vi "Read Provided Interface.vi"(8 "error in (no error)":errorcluster, 11 "instrument in":refnum<class "Instrument.lvclass">) -> (0 "error out":errorcluster, 2 "provided interface":string, 3 "instrument out":refnum<class "Instrument.lvclass">)   [LabVIEW 2020, in "MeasurementLink Instrument.lvlib" / "Instrument.lvclass"]
doc: "Returns the provided interface that will be used to query the MeasurmentLink Discovery Service for the address and port of the instrument's gRPC server. If your instrument does not use a gRPC server then you do not have to implement this VI."
uses:
  Instrument.lvclass
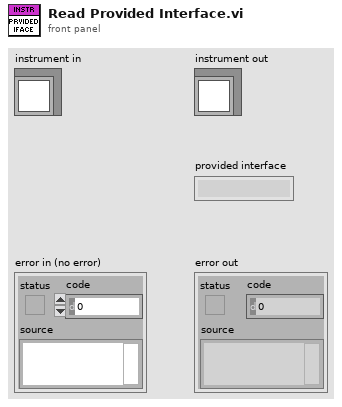
[diagram p1: front panel]
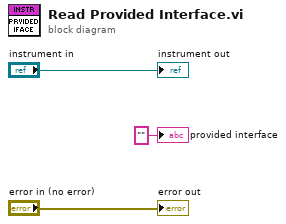
[diagram p0: block diagram]
diagram:
  "error out" <- "error in (no error)"
  "instrument out" <- "instrument in"
  "provided interface" <- "" ("grpc device interface")
